vi "Continuous Serial Write and Read.vi"() -> ()   [LabVIEW 2014]
doc: "This example performs writes and reads on a serial port, as directed by the user. You can press the Write and Read buttons, and change the Read Count, while the example is running.\n\nThe parameters set for the serial port must match the parameters of the connected instrument or device. In this example, the Read Count parameter specifies the number of bytes that the serial port reads. If there were more bytes at the port than the specified number, those bytes would not be read. If there were less bytes at the port than the specified number, you would receive a timeout error.\n\nThis example expands upon the flow control options for XON and XOFF, allowing the user to choose those control characters. Also, the user can enable or disable a termination character. Some devices require a termination character in order to identify the end of command strings. Some devices send a termination character to signify the end of data to be read. This example shows how you can end the Read operation once a termination character is detected in the buffer and/or append a termination character at the end of the Write data."
uses:
  support/Serial - Settings.ctl
  <vilib>/Instr/_visa.llb/VISA Configure Serial Port (Instr).vi
panel:
  in  "indice1":u16
  in  "indice0":u16
  out "element 2":u8
  out "element":u8
  out "distance":u16
  in  "byte count":u32
  out "error out":errorcluster
  in  "Stop":bool
  in  "Read":bool
  in  "Serial Settings":T1={"baud rate"=9600, "data bits"=8, "parity"=enum."None", "stop bits"=10, "flow control"=0} {"flow control" items=["None"=0, "XON/XOFF"=1, "RTS/CTS"=2, "DTR/DSR"=4]; "stop bits" items=["1.0"=10, "1.5"=15, "2.0"=20]; "data bits" min=5 max=8 step=1; "baud rate" items=["75"=75, "110"=110, "134"=134, "150"=150, "300"=300, "600"=600, "1200"=1200, "1800"=1800, "2400"=2400, "4800"=4800, "7200"=7200, "9600"=9600, "14400"=14400, "19200"=19200, "28800"=28800, "38400"=38400, "56000"=56000, "57600"=57600, "115200"=115200, "128000"=128000, "230400"=230400]}
  in  "VISA resource name":refnum<visa-resource-name>="COM1"
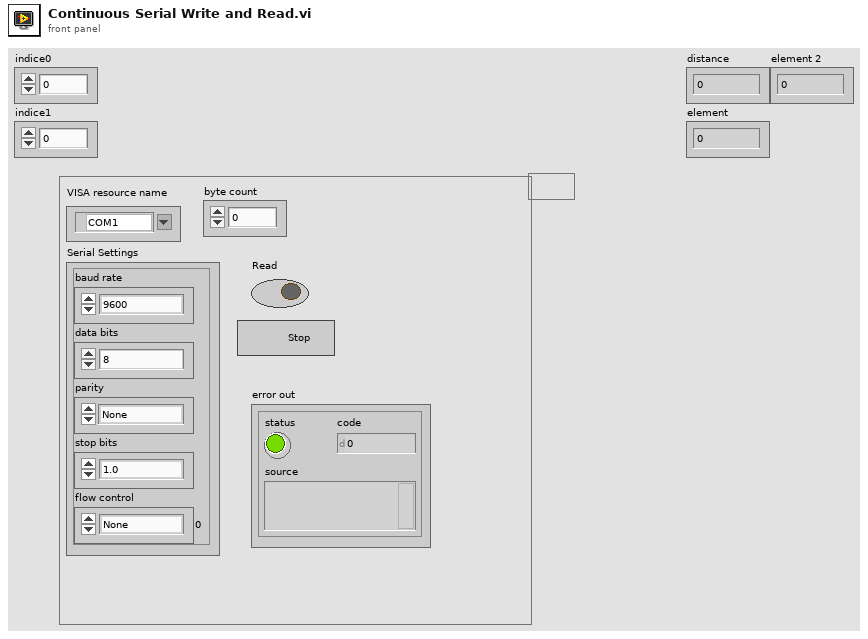
[diagram p1: front panel]
types:
  T1 = typedef "Serial - Settings.ctl" = cluster{"baud rate":u32, "data bits":u16, "parity":enum16{"None", "Odd", "Even", "Mark", "Space"}, "stop bits":u16, "flow control":u16}
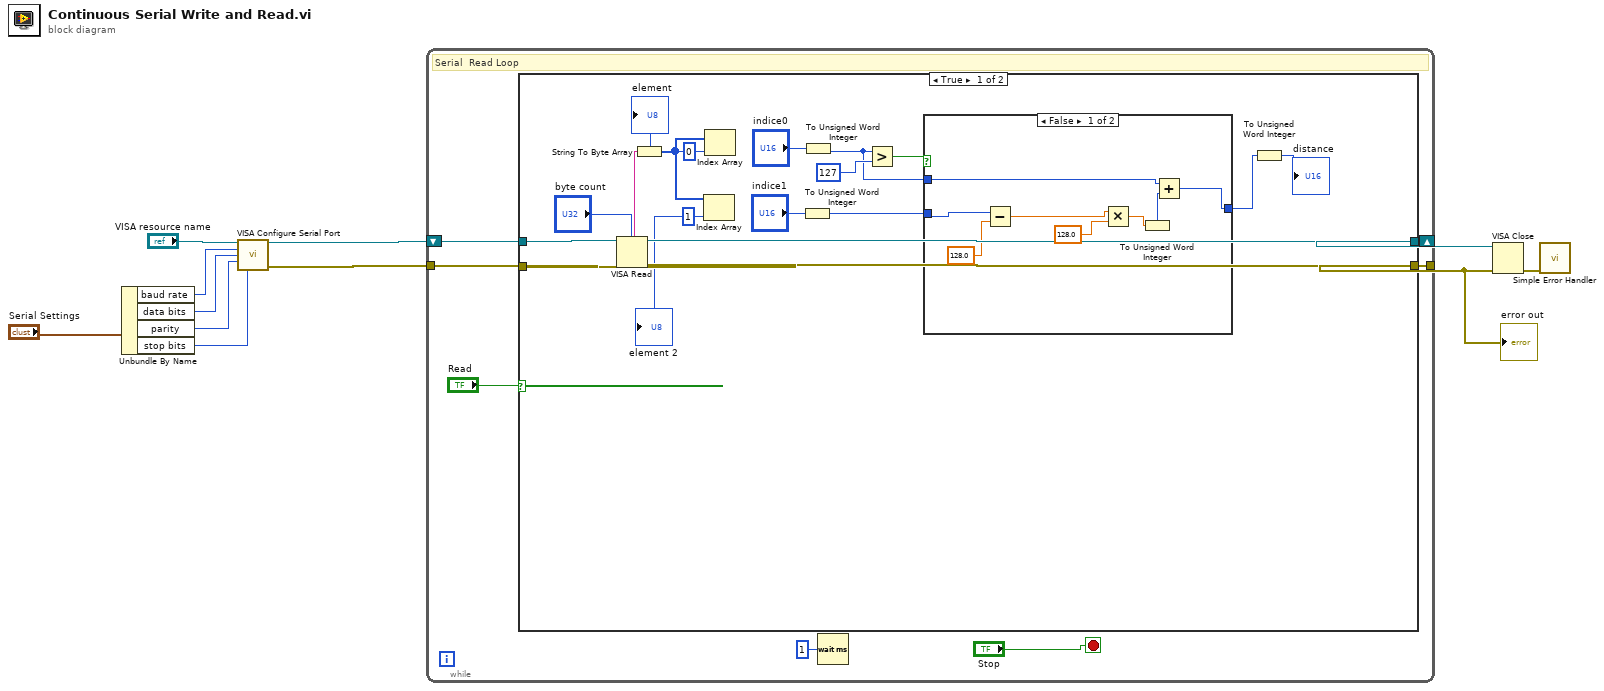
[diagram p0: block diagram]
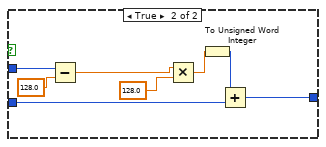
[diagram p2: hidden frame]
diagram:
  n1 = Unbundle By Name("Serial Settings") -> ("baud rate"=w7:u32, "data bits"=w8:u16, "parity"=w9:enum16{"None", "Odd", "Even", "Mark", "Space"}, "stop bits"=w10:u16)
  n2 = call-poly "VISA Configure Serial Port"("VISA resource name"="VISA resource name", "baud rate (9600)"=w7, "data bits (8)"=w8, "parity (0:none)"=w9, "stop bits (10: 1 bit)"=w10) -> ("VISA resource name out"=w4:refnum<visa-resource-name>, "error out"=w2:errorcluster)  [unwired: 5 in, 4 out]
  n3 = while {
    shift-right: [w18] -> w5
    shift-left: w4 -> [w14]
    tunnel: w2 -> [w15]
    tunnel: [w13] -> w3
    stop <- "Stop" stop-if-true
    # "Serial  Read Loop"
    n4 = case shown="True" "Read" {
      tunnel: [w35 w55] -> w18
      tunnel: w14 -> [w37 w55]
      tunnel: [w33 w54] -> w13
      tunnel: w15 -> [w36 w54]
      frame True {
        n5 = VISA Read(VISA resource name=w37, byte count="byte count", error in (no error)=w36) -> (VISA resource name out=w35:refnum<visa-resource-name>, read buffer=w25:string, error out=w33:errorcluster)  [unwired: 1 out]
        n6 = String To Byte Array(string=w25) -> (unsigned byte array=w32:u8[])
        n7 = Index Array(array=w32, index=1) -> (element=→"element 2":u8)
        n8 = Index Array(array=w32, index=0) -> (element=→"element":u8)
        n9 = To Unsigned Word Integer(number="indice1") -> (unsigned 16bit integer=w26:u16)
        n10 = To Unsigned Word Integer(number="indice0") -> (unsigned 16bit integer=w27:u16)
        n11 = Greater?(x=w27, y=u16 127) -> (0:w28:bool)
        n12 = case shown="False" w28 {
          tunnel: w27 -> [w41 w51]
          tunnel: w26 -> [w42 w49]
          tunnel: [w40 w48] -> w24
          frame False {
            n13 = Subtract(x=w42, y=128.0) -> (x-y=w43:dbl)
            n14 = Multiply(x=w43, y=128.0) -> (x*y=w39:dbl)
            n15 = To Unsigned Word Integer(number=w39) -> (unsigned 16bit integer=w38:u16)
            n16 = Add(x=w41, y=w38) -> (x+y=w40:u16)
          }
          frame True {
            n17 = Subtract(x=w51, y=128.0) -> (x-y=w50:dbl)
            n18 = Multiply(x=w50, y=128.0) -> (x*y=w47:dbl)
            n19 = To Unsigned Word Integer(number=w47) -> (unsigned 16bit integer=w46:u16)
            n20 = Add(x=w46, y=w49) -> (x+y=w48:u16)
          }
        }
        n21 = To Unsigned Word Integer(number=w24) -> (unsigned 16bit integer=→"distance":u16)
      }
      frame False {
      }
    }
    n22 = Wait (ms)(milliseconds to wait=u32 1) -> ()  [unwired: 1 out]
  }
  "error out" <- w3
  n23 = VISA Close(VISA resource name=w5, error in (no error)=w3) -> (error out=w6:errorcluster)
  n24 = call <vilib>:"Simple Error Handler.vi"("error in (no error)"=w6) -> ()  [unwired: 1 in, 8 out]
